vi "题目8.vi"() -> ()   [LabVIEW 2017]
panel:
  out "y":dbl
  in  "n":i32
  in  "m":i32
  in  "x":i32
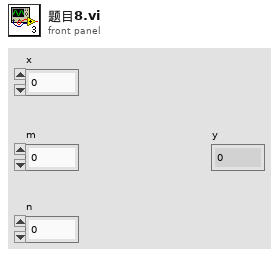
[diagram p1: front panel]
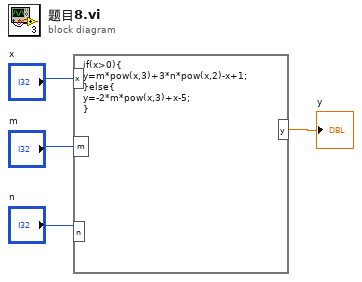
[diagram p0: block diagram]
diagram:
  n1 = formula code="if(x>0){\ny=m*pow(x,3)+3*n*pow(x,2)-x+1;\n}else{\ny=-2*m*pow(x,3)+x-5;\n}"("x"="x", "m"="m", "n"="n") -> ("y"=→"y":dbl)
